vi "9770 Filter ENB.vi"(10 "Frequency Spacing":dbl, 11 "Half  BW":dbl) -> (3 "ENB":dbl)   [LabVIEW 2017, in "EmsaAnalysis.lvlib"]
uses:
  <vilib>/addons/InsightCM/Devices/Shared/Emsa/EmsaAnalysis/EmsaAnalysis.lvlib
  <vilib>/Analysis/1siggen.llb/Ramp Pattern by Delta.vi
  <vilib>/addons/Digital Filter Design/NI_DigFilterLicensed.lvlib
  <vilib>/Analysis/NI_AALBase.lvlib
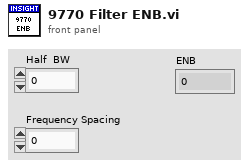
[diagram p1: front panel]
types:
  T1 = enum16{"Lowpass", "Highpass", "Bandpass", "Bandstop"}
  T2 = typedef "NI_DigFilterLicensed.lvlib/DFD Filter Obj.ctl" = cluster{"mSRate_Fs":dbl, "mSRate_Version":string, "mSRate_Comments":string, "mSRate_OrgCoef":T3, "mSRate_CurCoef":T3, "mSRate_Quantized?":bool, "mSRate_QCoef":T3, "mSRate_QSettings":T5[], "mSRate_Order":i32, "mSRate_Scaling":cluster{"mSRate_ScaleByPowerOf2?":bool, "mSRate_ScaleType":T7}}
  T3 = typedef "NI_DigFilterLicensed.lvlib/DFD Filter Coef.ctl" = cluster{"type":T4, "gain":dbl, "coef a (k)":dbl[], "coef b (v)":dbl[]}
  T4 = typedef "NI_DigFilterLicensed.lvlib/DFD Filter Structure Type Selector.ctl" = enum16{"Undefined", "FIR Direct Form", "FIR Direct Form Transposed", "FIR Symmetric", "FIR Antisymmetric", "IIR Direct Form I", "IIR Direct Form I Transposed", "IIR Direct Form II", "IIR Direct Form II Transposed", "IIR Cascaded Second Order Sections Form I", "IIR Cascaded Second Order Sections Form I Transposed", "IIR Cascaded Second Order Sections Form II", "IIR Cascaded Second Order Sections Form II Transposed", "Lattice Allpass (basic sections)", "Lattice Allpass (one multiplier sections)", "Lattice Allpass (normalized sections)", "Lattice AR (basic sections)", "Lattice AR (one multiplier sections)", "Lattice AR (normalized sections)", "Lattice MA (minimum phase)", "Lattice MA (maximum phase)", "Lattice ARMA (basic sections)", "Lattice ARMA (one multiplier sections)", "Lattice ARMA (normalized sections)"}
  T5 = typedef "NI_DigFilterLicensed.lvlib/dfd_Internal Quantization Settings.ctl" = cluster{"source":T6, "wl":i16, "iwl":i16, "overflow mode":enum16{"Saturation", "Wrap"}, "rounding mode":enum16{"Nearest", "Truncation"}, "signed?":bool}
  T6 = typedef "NI_DigFilterLicensed.lvlib/dfd_Internal Quantization Srcs.ctl" = u16
  T7 = typedef "NI_DigFilterLicensed.lvlib/DFD Coef Norm Type.ctl" = enum16{"No Norm", "Time Domain 1-Norm", "Time Domain 2-Norm", "Time Domain Inf-Norm"}
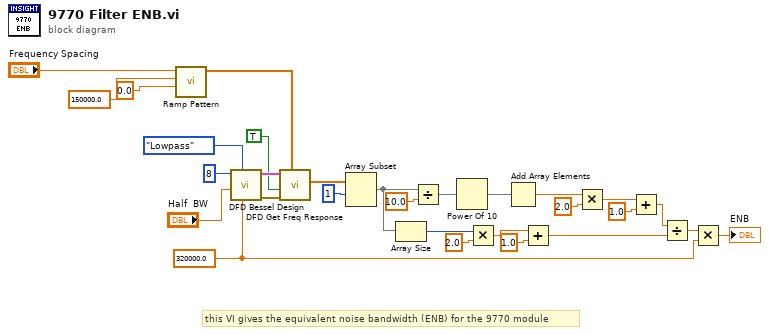
[diagram p0: block diagram]
diagram:
  w1 = 320000.0 ("sampling freq: fs")
  # "this VI gives the equivalent noise bandwidth (ENB) for the 9770 module"
  n1 = call-poly <vilib>:"Ramp Pattern.vi"("start"=0.0, "end"=150000.0, "delta"="Frequency Spacing") -> ("Ramp Pattern"=w23:dbl[])  [unwired: 6 in, 2 out]
  n2 = call <vilib>:"DFD Bessel Design.vi"("fs [Hz]"=w1, "filter type"=T1."Lowpass", "low cutoff freq [Hz]"="Half  BW", "order"=8) -> ("error out"=w26:errorcluster, "filter out"=w28:T2)  [unwired: 6 in]
  n3 = call <vilib>:"DFD Get Freq Response.vi"("freq points [Hz]"=w23, "error in (no error)"=w26, "dB on? (T)"=TRUE, "filter in"=w28) -> ("magnitude"=w19:dbl[])  [unwired: 4 in, 3 out]
  n4 = Array Subset(array=w19, index=1) -> (w8:dbl[])  [unwired: 1 in]
  n5 = Array Size(array=w8) -> (size(s)=w7:i32)
  n6 = Divide(x=w8, y=10.0) -> (x/y=w20:dbl[])
  n7 = Power Of 10(x=w20) -> (10^x=w2:dbl[])
  n8 = Multiply(x=w7, y=2.0) -> (x*y=w11:dbl)
  n9 = Add Array Elements(numeric array=w2) -> (sum=w16:dbl)
  n10 = Add(x=w11, y=1.0) -> (x+y=w9:dbl)
  n11 = Multiply(x=w16, y=2.0) -> (x*y=w15:dbl)
  n12 = Add(x=w15, y=1.0) -> (x+y=w13:dbl)
  n13 = Divide(x=w13, y=w9) -> (x/y=w6:dbl)
  n14 = Multiply(x=w6, y=w1) -> (x*y=→"ENB":dbl)
